vi "Target Mode.vi"() -> ()   [LabVIEW 2019, in "Inst.MOTOR.lvclass"]
uses:
  Inst.MOTOR.lvclass
panel:
  in  "Speed":i32
  in  "Target Position":i32
  out "Inst.MOTOR out":refnum<class "Inst.MOTOR.lvclass">
  out "read buffer":string
  out "error out":errorcluster
  in  "Inst.MOTOR in":refnum<class "Inst.MOTOR.lvclass">
  in  "error in (no error)":errorcluster
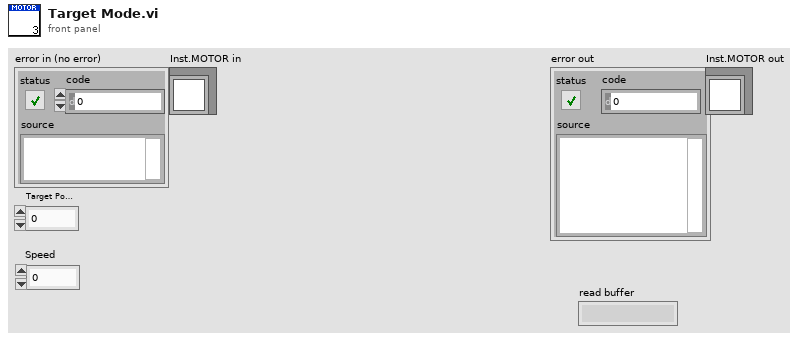
[diagram p1: front panel]
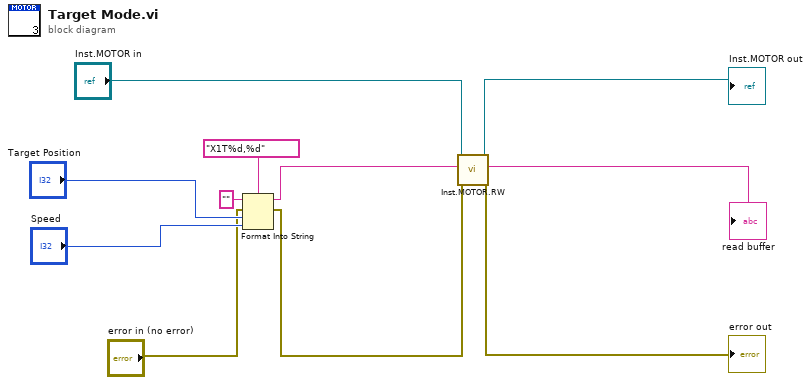
[diagram p0: block diagram]
diagram:
  n1 = Format Into String(format string="X1T%d,%d", initial string="", error in="error in (no error)", "Target Position", "Speed") -> (resulting string=w6:string, error out=w2:errorcluster)
  n2 = call "Inst.MOTOR.RW.vi"("error in (no error)"=w2, "Data in"=w6, "Inst.MOTOR in"="Inst.MOTOR in") -> ("error out"=→"error out":errorcluster, "read buffer"=→"read buffer":string, "Inst.MOTOR out"=→"Inst.MOTOR out":refnum<class "Inst.MOTOR.lvclass">)  [unwired: 6 in]
